vi "Tom_Dialog.vi"(5 "error in (no error)":errorcluster) -> (16 "Name out":string, 17 "OK":bool)   [LabVIEW 2024]
doc: "Displays a standard dialog box that prompts users to enter information, such as a user name and password.\n--------------------\n\nThis Express VI is configured as follows:\n\nMessage to Display to the User:hkjh jkl \nThe inputs are: \nText Entry Box: test"
panel:
  in  "Input Name":string="test"
  out "error out":errorcluster
  in  "Cancel":bool
  in  "OK2":bool
  # "Enter the name of your new instrument folder"
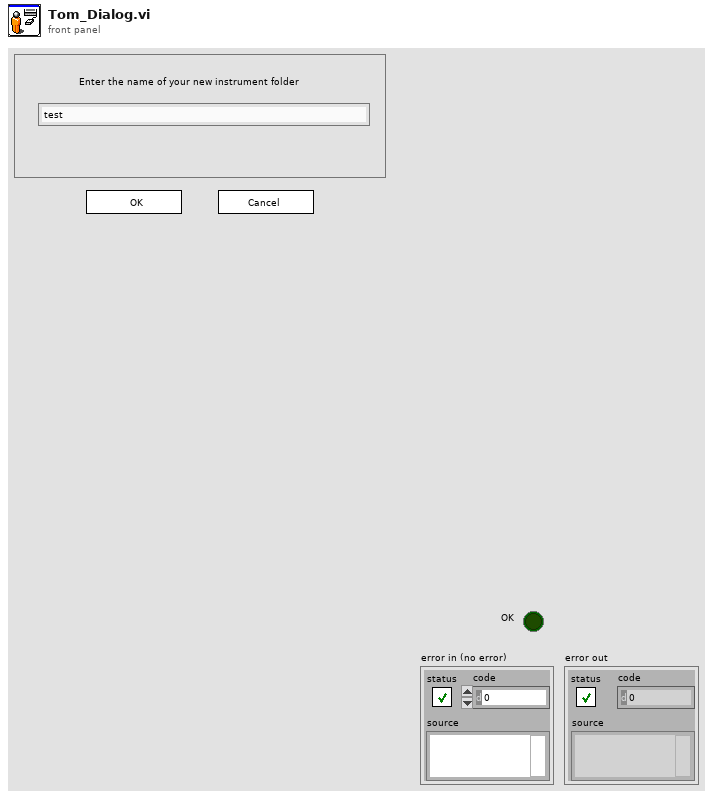
[diagram p1: front panel]
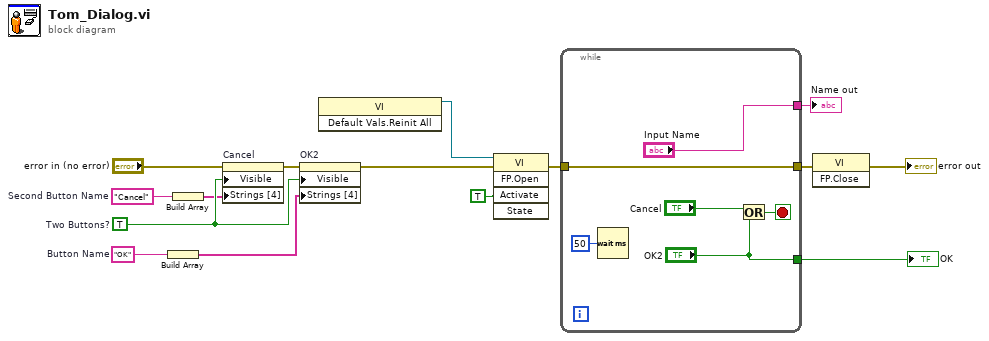
[diagram p0: block diagram]
diagram:
  w11 = "Cancel"  # Second Button Name
  w9 = "OK"  # Button Name
  w15 = TRUE  # Two Buttons?
  n1 = Build Array(w9) -> (w10:string[])
  n2 = Build Array(w11) -> (w12:string[])
  n3 = property on="Cancel" class="Bool"(error in="error in (no error)", "Visible"=w15, "Strings [4]"=w12) -> (error out=w13:errorcluster)  [unwired: 1 in, 1 out]
  n4 = property on="OK2" class="Bool"(error in=w13, "Visible"=w15, "Strings [4]"=w10) -> (error out=w1:errorcluster)  [unwired: 1 in, 1 out]
  n5 = invoke class="VI" method="Default Vals.Reinit All"() -> (reference out=w6:refnum<vi>)  [unwired: 3 in, 2 out]
  n6 = invoke class="VI" method="FP.Open"(reference=w6, error in=w1, "Activate"=TRUE ("Activate?")) -> (error out=w4:errorcluster)  [unwired: 2 in, 4 out]
  n7 = while "Main While Loop" {
    tunnel: ["OK2"] -> w14
    tunnel: w4 -> [w18]
    tunnel: [w18] -> w3
    tunnel: ["Input Name"] -> w2
    stop <- w19 stop-if-true
    n8 = Wait (ms)(milliseconds to wait=u32 50 ("millisecond multiple")) -> ()  [unwired: 1 out]
    n9 = Or(x="Cancel", y="OK2") -> (x .or. y?=w19:bool)
  }
  "OK" <- w14
  "Name out" <- w2
  n10 = invoke class="VI" method="FP.Close"(error in=w3) -> (error out=→"error out":errorcluster)  [unwired: 2 in, 2 out]
